vi "Write Pattern.vi"(8 "error in (no error)":errorcluster, 10 "Pattern":enum16{"Rows", "Spiral"}(ring), 11 "Grid Animation in":refnum<class "Grid Animation.lvclass">) -> (0 "error out":errorcluster, 3 "Grid Animation out":refnum<class "Grid Animation.lvclass">)   [LabVIEW 2024, in "Grid Animation.lvlib" / "Grid Animation.lvclass"]
uses:
  Grid Animation.lvclass
  Grid Animation.lvclass/Grid Animation.ctl
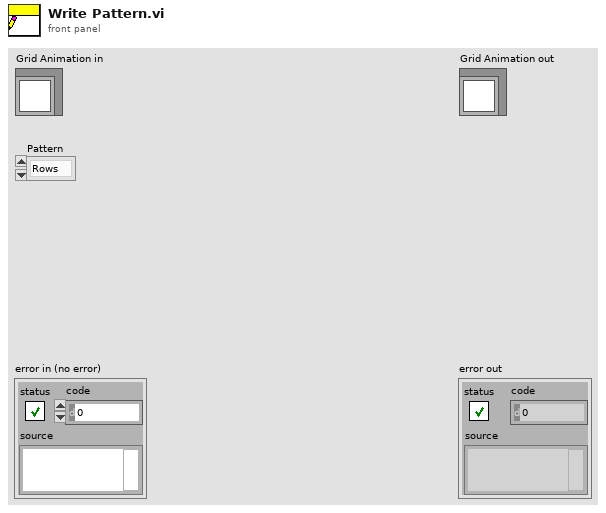
[diagram p1: front panel]
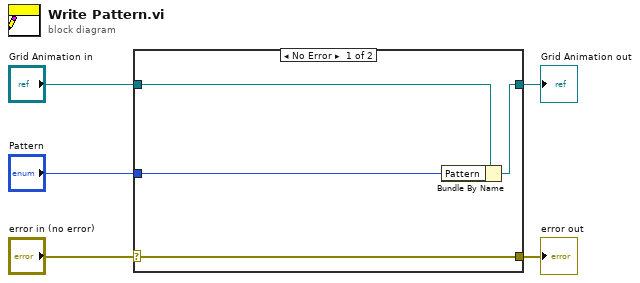
[diagram p0: block diagram]
diagram:
  n1 = case shown="No Error" "error in (no error)" {
    selector: "error in (no error)" -> [w9 w10]
    tunnel: [w9 w10] -> w4
    tunnel: [w7 w11] -> w2
    tunnel: "Grid Animation in" -> [w8 w11]
    tunnel: "Pattern" -> [w6 _]
    frame No Error {
      n2 = Bundle By Name(cluster=w8, "Pattern"=w6) -> (w7:refnum<class "Grid Animation.lvclass">)
    }
    frame Error {
    }
  }
  "error out" <- w4
  "Grid Animation out" <- w2
